vi "Filtro.vi"(11 "name or relative path 2":path=path "C:/Users/axel2/OneDrive/Documents/Ejercicios_Labview/Topicos Selectos/Proyecto/Ex3_ComSerial_Ard_LV/mexico_tmo_2013066_lrg.jpg") -> (0 "Área de particulas":T1(graph), 1 "ROJO":bool, 2 "AMBAR":bool, 3 "VERDE":bool, 4 "Original 2":T4(plugin-control) caption="Original Image", 5 "Área de particualas total":dbl, 7 "Number of Particles 2":i32, 10 "Particle Reports (Real-World)":T2(array[cluster]) {"Orientation" format="%.2f"; "Dimensions"."Height" format="%.2f"; "Dimensions"."Width" format="%.2f"; "Center of Mass"."Y" format="%.2f"; "Center of Mass"."X" format="%.2f"; "Bounding Rect"."Bottom" format="%.2f"; "Bounding Rect"."Right" format="%.2f"; "Bounding Rect"."Top" format="%.2f"; "Bounding Rect"."Left" format="%.2f"; "Number of Holes" format="%.2f"; "Area" format="%.2f"})   [LabVIEW 2020]
doc: "This example performs a series of grayscale filtering, threshold, binary morphology, and particle analysis operations to measure the areas of all the large circular particles of the image."
uses:
  <vilib>/vision/NI_Vision_Development_Module.lvlib
panel:
  in  "Tab Control 2":T3(tab)
  out "Threshold 2":T4(plugin-control) caption="Threshold Image"
  out "Fill Hole and Reject Border 2":T4(plugin-control) caption="Reject Border and Fill Holes"
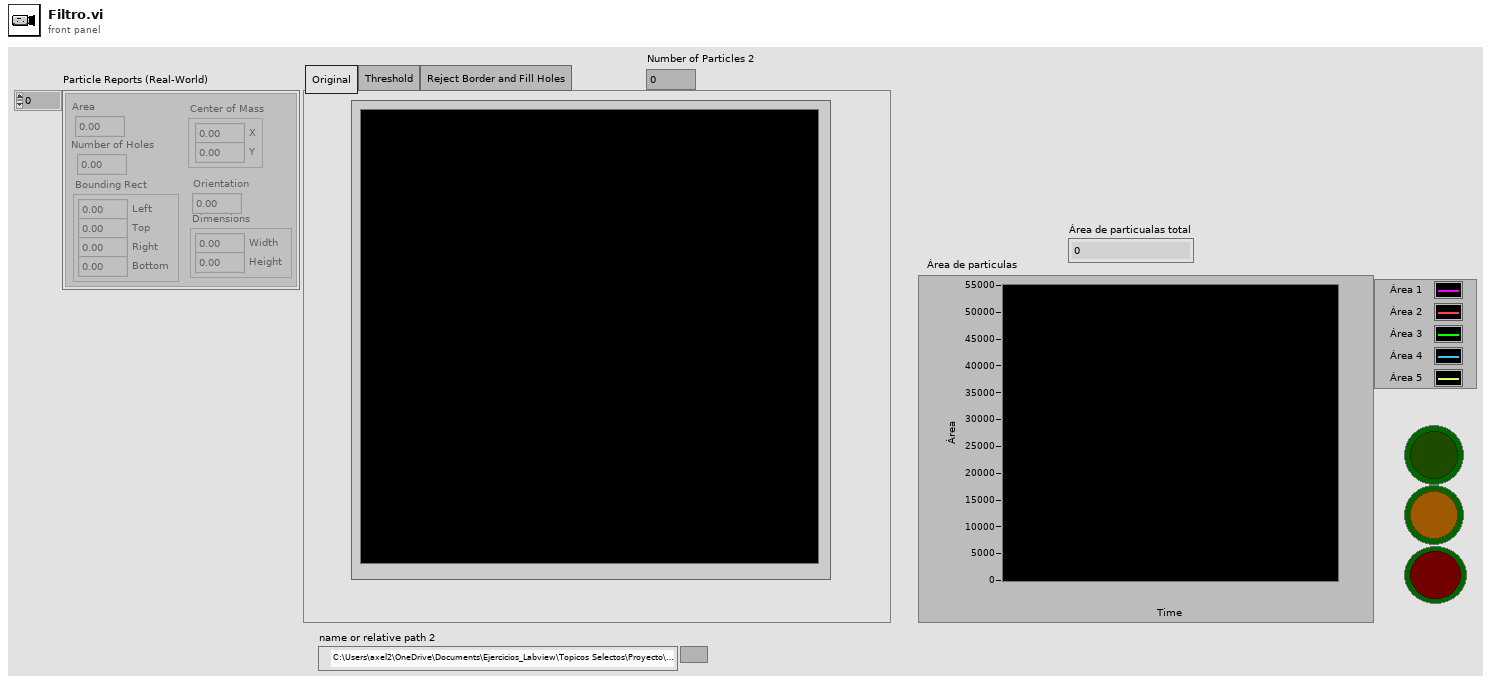
[diagram p1: front panel]
types:
  T1 = cluster{"Area":dbl, "Area":dbl, "Area":dbl, "Area":dbl, "Area":dbl, "Area":dbl}
  T2 = cluster{"Area":dbl, "Number of Holes":dbl, "Bounding Rect":cluster{"Left":dbl, "Top":dbl, "Right":dbl, "Bottom":dbl}, "Center of Mass":cluster{"X":dbl, "Y":dbl}, "Orientation":dbl, "Dimensions":cluster{"Width":dbl, "Height":dbl}}[]
  T3 = enum32{"Original", "Threshold", "Reject Border and Fill Holes"}
  T4 = typedef "IMAQ Image.ctl" = refnum<image>
  T5 = typedef "Image Type" = u32
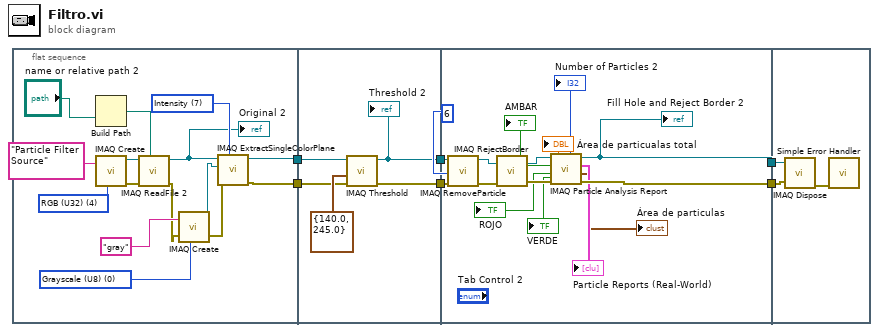
[diagram p0: block diagram]
diagram:
  n1 = flat-sequence {
    tunnel: [w9] -> w6
    tunnel: [w16] -> w5
    tunnel: [w24] -> w4
    tunnel: [w25] -> w3
    tunnel: w6 -> [w23]
    tunnel: w5 -> [w22]
    tunnel: w4 -> [w42]
    tunnel: w3 -> [w41]
    tunnel: [w33] -> w2
    tunnel: [w35] -> w1
    tunnel: w2 -> [w44]
    tunnel: w1 -> [w43]
    frame #0 {
      w13 = T5 0 items=["Grayscale (U8)", "Grayscale (I16)", "Grayscale (SGL)", "Complex (CSG)", "RGB (U32)", "HSL (U32)", "RGB (U64)", "Grayscale (U16)"] ("Image Type")
      w15 = 7 items=["Red", "Green", "Blue", "Hue", "Saturation", "Luminance", "Value", "Intensity"] ("Color Plane")
      w17 = T5 4 items=["Grayscale (U8)", "Grayscale (I16)", "Grayscale (SGL)", "Complex (CSG)", "RGB (U32)", "HSL (U32)", "RGB (U64)", "Grayscale (U16)"] ("Image Type")
      n2 = Build Path(name or relative path="name or relative path 2") -> (appended path=w21:path)  [unwired: 1 in]
      n3 = call "IMAQ Create"("Image Name"="Particle Filter Source", "Image Type"=w17) -> ("New Image"=w19:T4, "error out"=w18:errorcluster)  [unwired: 3 in]
      n4 = call "IMAQ ReadFile 2"("File Path"=w21, "error in (no error)"=w18, "Image"=w19) -> ("error out"=w11:errorcluster, "Image Out"=w8:T4)  [unwired: 4 in, 3 out]
      "Original 2" <- w8
      n5 = call "IMAQ Create"("Image Name"="gray", "Image Type"=w13, "error in (no error)"=w11) -> ("New Image"=w14:T4, "error out"=w10:errorcluster)  [unwired: 2 in]
      n6 = call "IMAQ ExtractSingleColorPlane"("Color Plane"=w15, "error in (no error)"=w10, "Image Dst"=w14, "Image Src"=w8) -> ("error out"=w16:errorcluster, "Image Dst Out"=w9:T4)  [unwired: 6 in]
    }
    frame #1 {
      n7 = call "IMAQ Threshold"("error in (no error)"=w22, "Range"=cluster{"Lower value":sgl, "Upper value":sgl} {"Lower value"=140.0, "Upper value"=245.0}, "Image Src"=w23) -> ("error out"=w25:errorcluster, "Image Dst Out"=w24:T4)  [unwired: 7 in]
      "Threshold 2" <- w24
    }
    frame #2 {
      n8 = call "IMAQ RemoveParticle"("error in (no error)"=w41, "Number of Erosion"=6, "Image Src"=w42) -> ("error out"=w39:errorcluster, "Image Dst Out"=w40:T4)  [unwired: 7 in]
      n9 = call "IMAQ RejectBorder"("error in (no error)"=w39, "Image Src"=w40) -> ("error out"=w36:errorcluster, "Image Dst Out"=w37:T4)  [unwired: 4 in]
      n10 = call "IMAQ Particle Analysis Report"("error in (no error)"=w36, "Image"=w37) -> ("error out"=w35:errorcluster, "output cluster"=→"Área de particulas":T1, "Particle Reports (Real-World)"=→"Particle Reports (Real-World)":T2, "Image Out (duplicate)"=w33:T4, "Number of Particles"=→"Number of Particles 2":i32, "VERDE"=→"VERDE":bool, "Área de particualas total"=→"Área de particualas total":dbl, "ROJO"=→"ROJO":bool, "AMBAR"=→"AMBAR":bool)  [unwired: 1 out]
      "Fill Hole and Reject Border 2" <- w33
    }
    frame #3 {
      n11 = call "IMAQ Dispose"("Image"=w44, "error in (no error)"=w43) -> ("error out"=w45:errorcluster)  [unwired: 4 in]
      n12 = call <vilib>:"Simple Error Handler.vi"("error in (no error)"=w45) -> ()  [unwired: 4 in, 5 out]
    }
  }
